vi "Matrix Add and show result.vi"() -> ()   [LabVIEW 2014, in "Arduino MatrixMath.lvlib"]
uses:
  Arduino MatrixMath.lvlib
  <vilib>/LabVIEW Universal Transcriptor/LabVIEW for Arduino SoftwareSerial Library/Arduino SoftwareSerial Wrapper.lvlib
panel:
  in  "B":sgl[](array[numeric])=[1.0, 2.0, 3.0, 4.0, 5.0, 6.0, 7.0, 8.0]
  out "Error Out":errorcluster
  in  "Error In":errorcluster
  in  "A":sgl[](array[numeric])=[1.0, 2.0, 3.0, 4.0, 5.0, 6.0, 7.0, 8.0]
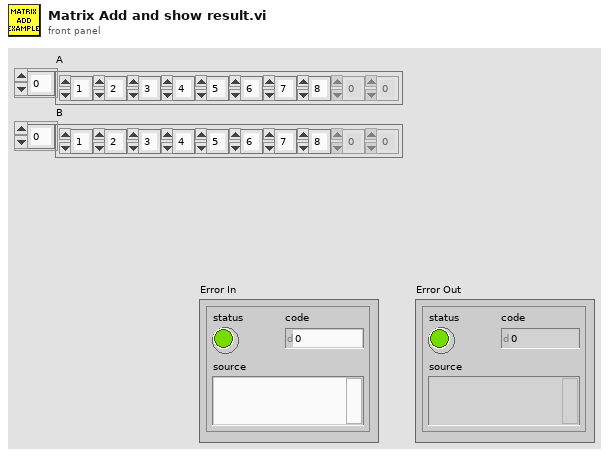
[diagram p1: front panel]
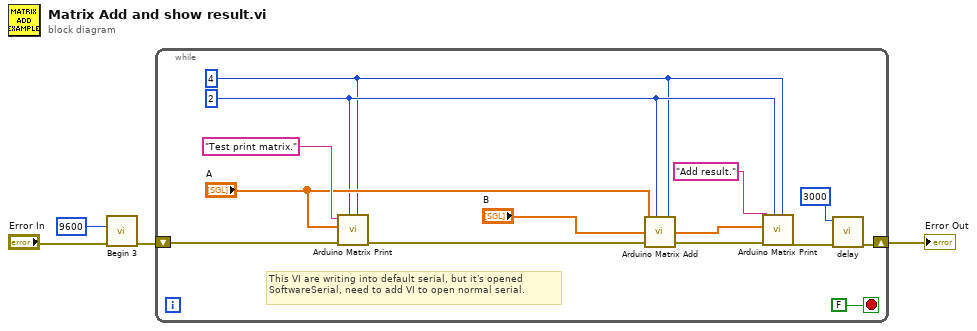
[diagram p0: block diagram]
diagram:
  n1 = call <vilib>:"Begin 3.vi"("Error In"="Error In", "Baudrate"=u32 9600 ("Speed")) -> ("Error Out"=w2:errorcluster)  [unwired: 8 in]
  n2 = while {
    shift-right: [w7] -> w4
    shift-left: w2 -> [w15]
    stop <- FALSE stop-if-true
    w8 = u8 4 ("cols num.")
    w9 = u8 2 ("rows num.")
    # "This VI are writing into default serial, but it's opened SoftwareSerial, need to add VI to open normal serial."
    n3 = call "Arduino Matrix Print.vi"("cols num."=w8, "rows num."=w9, "Error In"=w15, "A"="A", "Label"="Test print matrix.") -> ("Error Out"=w17:errorcluster)  [unwired: 6 in]
    n4 = call "Arduino Matrix Add.vi"("A"="A", "rows num."=w9, "B"="B", "Error In"=w17, "cols num."=w8) -> ("A+B"=w12:sgl[], "Error Out"=w13:errorcluster)  [unwired: 1 in]
    n5 = call "Arduino Matrix Print.vi"("cols num."=w8, "rows num."=w9, "Error In"=w13, "A"=w12, "Label"="Add result.") -> ("Error Out"=w6:errorcluster)  [unwired: 6 in]
    n6 = call <vilib>:"delay.vi"("Error In"=w6, "time (ms)"=3000) -> ("Error Out"=w7:errorcluster)  [unwired: 9 in]
  }
  "Error Out" <- w4
